vi "FRCts20_WebMethods_Redirect_Team.vi"(7 "response code (200)":i32(ring)=200 items=["100"=100, "101"=101, "200"=200, "201"=201, "202"=202, "203"=203, "204"=204, "205"=205, "206"=206, "300"=300, "301"=301, "302"=302, "303"=303, "304"=304, "305"=305, "306"=306, "307"=307, "400"=400, "401"=401, "402"=402, "403"=403, "404"=404, "405"=405, "406"=406, "407"=407, "408"=408, "409"=409, "410"=410, "411"=411, "412"=412, "413"=413, "414"=414, "415"=415, "416"=416, "417"=417, "500"=500, "501"=501, "502"=502, "503"=503, "504"=504, "505"=505], 8 "error in (no error)":errorcluster, 10 "Team":T1, 11 "httpRequestID":u32) -> (0 "error out":errorcluster, 3 "httpRequestID out":u32)   [LabVIEW 2014, in "FRCts20_WebMethods.lvlib"]
uses:
  FRCts20_WebMethods.lvlib
  Backend/source/VI Source/FRCts20_Backend_API/FRCts20_Backend_API_Team.ctl
  Backend/source/VI Source/FRCts20_Backend_API/FRCts20_Backend_API_SW.ctl
  Backend/source/VI Source/FRCts20_Backend_API/FRCts20_Backend_API_Status.ctl
  <vilib>/wsapi/NI_WebServices.lvlib
  Backend/source/VI Source/FRCts20_Backend_API/FRCts20_Backend_API.lvlib
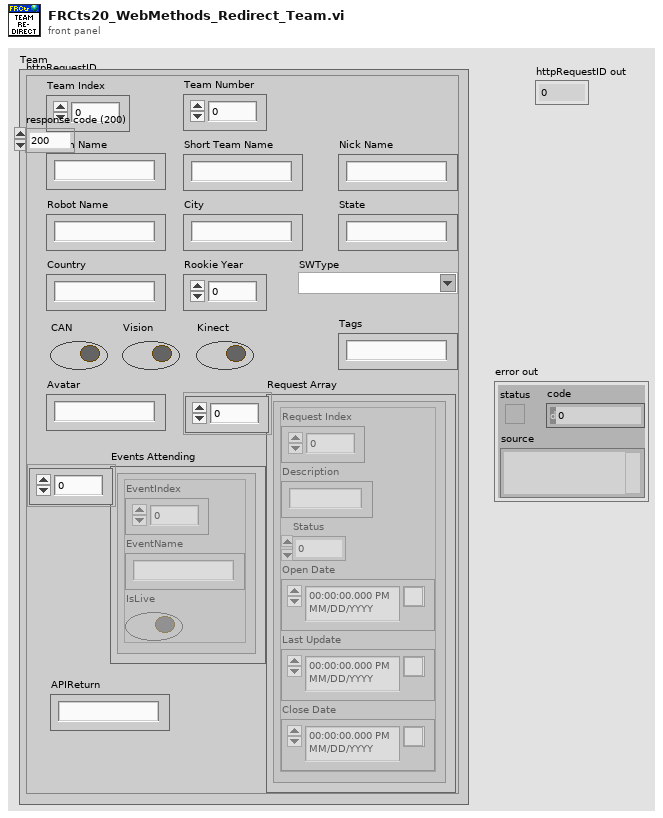
[diagram p1: front panel]
types:
  T1 = typedef "FRCts20_Backend_Engine.lvlib/FRCts20_Backend_API.lvlib/FRCts20_Backend_API_Team.ctl" = cluster{"Team Index":u32, "Team Number":u32, "Team Name":string, "Short Team Name":string, "Nick Name":string, "Robot Name":string, "City":string, "State":string, "Country":string, "Rookie Year":u32, "SWType":T2, "CAN":bool, "Vision":bool, "Kinect":bool, "Tags":string, "Avatar":string, "Request Array":cluster{"Request Index":u32, "Description":string, "Status":T3, "Open Date":timestamp, "Last Update":timestamp, "Close Date":timestamp}[], "Events Attending":cluster{"EventIndex":i32, "EventName":string, "IsLive":bool}[], "APIReturn":string}
  T2 = typedef "FRCts20_Backend_Engine.lvlib/FRCts20_Backend_API.lvlib/FRCts20_Backend_API_SW.ctl" = string
  T3 = typedef "FRCts20_Backend_Engine.lvlib/FRCts20_Backend_API.lvlib/FRCts20_Backend_API_Status.ctl" = i32
  T4 = typedef "FRCts20_WebMethods.lvlib/FRCts20_WebMethods_ctl_returntype.ctl" = string
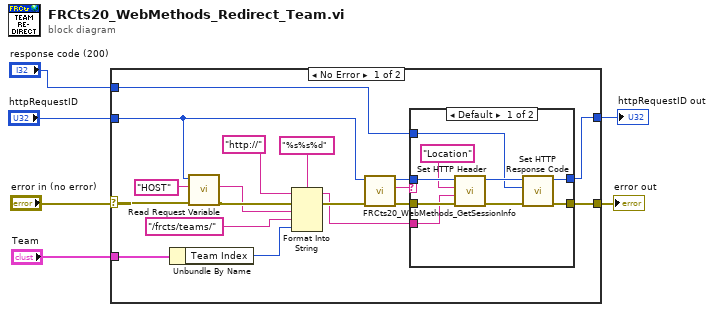
[diagram p0: block diagram]
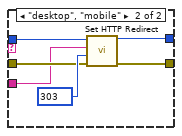
[diagram p2: hidden frame]
diagram:
  n1 = case shown="No Error" "error in (no error)" {
    selector: "error in (no error)" -> [w11 w41]
    tunnel: [w15 w41] -> w6
    tunnel: "httpRequestID" -> [w7 w40]
    tunnel: [w14 w40] -> w4
    tunnel: "Team" -> [w24 _]
    tunnel: "response code (200)" -> [w12 _]
    frame No Error {
      n2 = Unbundle By Name(w24) -> ("Team Index"=w20:u32)
      n3 = call <vilib>:"Read Request Variable.vi"("error in (no error)"=w11, "variable name"="HOST", "httpRequestID"=w7) -> ("error out"=w10:errorcluster, "value"=w9:string)  [unwired: 6 in, 1 out]
      n4 = Format Into String(format string="%s%s%d", initial string="http://", error in=w10, w9, "/frcts/teams/", w20) -> (resulting string=w13:string, error out=w16:errorcluster)
      n5 = call "FRCts20_WebMethods_GetSessionInfo.vi"("error in"=w16, "httpRequestID"=w7) -> ("error out"=w18:errorcluster, "Return Type"=w19:T4, "httpRequestID out"=w17:u32)  [unwired: 7 in]
      n6 = case shown="Default" w19 {
        tunnel: [w29 w39] -> w15
        tunnel: [w26 w38] -> w14
        tunnel: w18 -> [w33 w36]
        tunnel: w17 -> [w32 w35]
        tunnel: w13 -> [w30 w34]
        tunnel: w12 -> [w25 _]
        frame Default {
          n7 = call <vilib>:"Set HTTP Header.vi"("error in (no error)"=w33, "header value"=w30, "header"="Location", "httpRequestID"=w32) -> ("error out"=w28:errorcluster, "httpRequestID out"=w27:u32)  [unwired: 6 in]
          n8 = call <vilib>:"Set HTTP Response Code.vi"("error in (no error)"=w28, "response code (200)"=w25, "httpRequestID"=w27) -> ("error out"=w29:errorcluster, "httpRequestID out"=w26:u32)  [unwired: 7 in]
        }
        frame "desktop", "mobile" {
          w37 = 303 items=["100"=100, "101"=101, "200"=200, "201"=201, "202"=202, "203"=203, "204"=204, "205"=205, "206"=206, "300"=300, "301"=301, "302"=302, "303"=303, "304"=304, "305"=305, "306"=306, "307"=307, "400"=400, "401"=401, "402"=402, "403"=403, "404"=404, "405"=405, "406"=406, "407"=407, "408"=408, "409"=409, "410"=410, "411"=411, "412"=412, "413"=413, "414"=414, "415"=415, "416"=416, "417"=417, "500"=500, "501"=501, "502"=502, "503"=503, "504"=504, "505"=505] ("response code (307)")
          n9 = call <vilib>:"Set HTTP Redirect.vi"("error in (no error)"=w36, "response code (307)"=w37, "redirect URL"=w34, "httpRequestID"=w35) -> ("error out"=w39:errorcluster, "httpRequestID out"=w38:u32)  [unwired: 6 in]
        }
      }
    }
    frame Error {
    }
  }
  "error out" <- w6
  "httpRequestID out" <- w4
